vi "Instrument.Aerotech.Read Configuration File.vi"(8 "error in (no error)":errorcluster, 11 "Instrument.Aerotech":refnum<class "Instrument.Aerotech.lvclass">) -> (0 "error out":errorcluster, 3 "Instrument.Aerotech out":refnum<class "Instrument.Aerotech.lvclass">)   [LabVIEW 2016, in "Instrument.Aerotech.lvclass"]
uses:
  Instrument.Aerotech.lvclass
  <userlib>/LevyLab/Levylab Instruments/SMOs/Configuration/Configuration.lvclass
  <userlib>/LevyLab/Levylab Instruments/SMOs/Instrument/Instrument.lvclass
  C:/Program Files (x86)/National Instruments/LabVIEW 2016/user.lib/LevyLab/Levylab Instruments/SMOs/Instrument/Instrument.lvclass
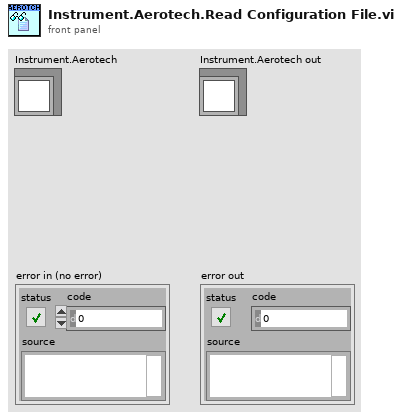
[diagram p1: front panel]
types:
  T1 = typedef "Instrument.Aerotech.lvclass/Instrument.Aerotech.Configuration--Cluster.ctl" = cluster{"Example Setting 1":dbl, "Example Setting 2":dbl, "Example Setting 3":string}
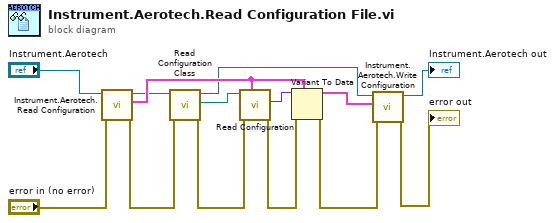
[diagram p0: block diagram]
diagram:
  n1 = call "Instrument.Aerotech.Read Configuration.vi"("error in (no error)"="error in (no error)", "Instrument.Aerotech"="Instrument.Aerotech") -> ("error out"=w6:errorcluster, "Configuration"=w10:T1, "Instrument.Aerotech out"=w8:refnum<class "Instrument.Aerotech.lvclass">)  [unwired: 7 in]
  n2 = call <userlib>:"Read Configuration Class.vi"("error in (no error)"=w6, "Instrument in"=w8) -> ("error out"=w5:errorcluster, "Configuration.lvclass"=w9:refnum<class "Configuration.lvclass">, "Instrument out"=w7:refnum<class "Instrument.Aerotech.lvclass">)  [unwired: 7 in]
  n3 = call <userlib>:"Read Configuration.vi"("INI Fomatted Cluster Type"=w10, "error in (no error)"=w5, "Configuration in"=w9) -> ("error out"=w13:errorcluster, "Configuration"=w14:variant)  [unwired: 6 in, 1 out]
  n4 = Variant To Data(error in=w13, type=w10, Variant=w14) -> (data=w12:T1, error out=w11:errorcluster)
  n5 = call "Instrument.Aerotech.Write Configuration.vi"("error in (no error)"=w11, "Configuration"=w12, "Instrument.Aerotech"=w7) -> ("error out"=→"error out":errorcluster, "Instrument.Aerotech out"=→"Instrument.Aerotech out":refnum<class "Instrument.Aerotech.lvclass">)  [unwired: 7 in]
